vi "FTW-Endpoint-Core-ResolveSymbol.vi"(8 "error in":errorcluster, 10 "Symbol":string) -> (0 "error out":errorcluster, 2 "Symbol Value":i32)   [LabVIEW 2013, in "FTW-Actor-Endpoint.lvclass"]
uses:
  FTW-Actor-Endpoint.lvclass
  FTW-Endpoint-Symbols.vi
panel:
  # "Inputs"
  # "Outputs"
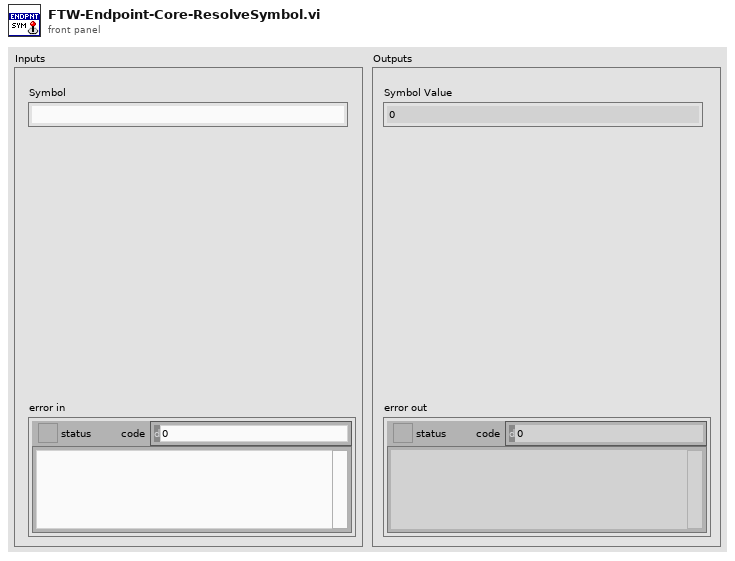
[diagram p1: front panel]
types:
  T1 = cluster{"Symbol Name":string, "Symbol Value":i32}[]
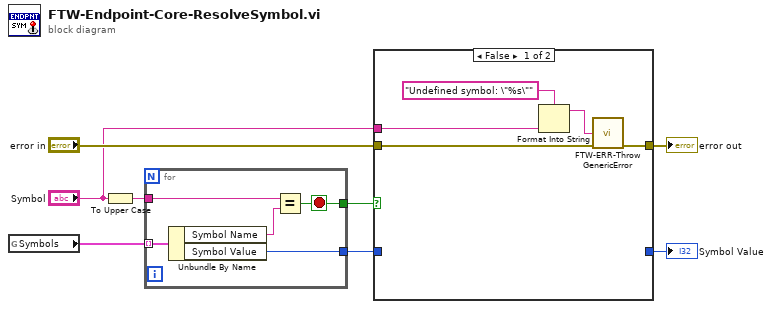
[diagram p0: block diagram]
diagram:
  n1 = global read "FTW-Endpoint-Symbols.vi" "Symbols"() -> (w8:T1)
  n2 = To Upper Case(1:"Symbol") -> (0:w7:string)
  n3 = for {
    tunnel: w8 -> [w13] mode=indexing
    tunnel: w7 -> [w11]
    tunnel: [w9] -> w1
    tunnel: [w10] -> w4
    stop <- w10 stop-if-true
    n4 = Unbundle By Name(w13) -> ("Symbol Name"=w12:string, "Symbol Value"=w9:i32)
    n5 = Equal?(x=w11, y=w12) -> (x = y?=w10:bool)
  }
  n6 = case shown="False" w4 {
    tunnel: [w17 w20] -> w6
    tunnel: "error in" -> [w18 w20]
    tunnel: "Symbol" -> [w16 _]
    tunnel: [_ w19] -> w2
    tunnel: w1 -> [_ w19]
    frame False {
      n7 = Format Into String(format string="Undefined symbol: \"%s\"", w16) -> (resulting string=w14:string)  [unwired: 2 in, 1 out]
      n8 = call "FTW-ERR-ThrowGenericError.vi"("Error Message"=w14, "error in"=w18) -> ("error out"=w17:errorcluster)  [unwired: 13 in]
    }
    frame True {
    }
  }
  "error out" <- w6
  "Symbol Value" <- w2
